vi "PNG Write.vi"(8 "error in (no error)":errorcluster, 10 "Chunks":T1[](array[typedef]) {"CRC" format="%08x"}, 11 "Image Path (*.png)":path) -> (0 "error out":errorcluster, 3 "dup Image Path":path)   [LabVIEW 2018, in "Export-Built-ins.lvlib"]
doc: "Writes the PNG image chunks to the <b>Image Path (*.png)</b>.\n\nCreated by: Ryan Pacini"
uses:
  Export-Built-ins.lvlib
  Controls/PNG Chunk.ctl
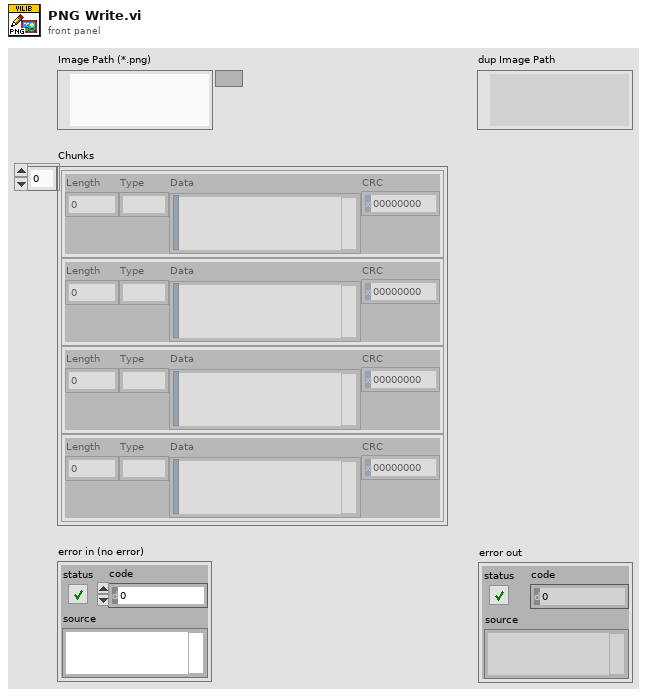
[diagram p1: front panel]
types:
  T1 = typedef "Export-Built-ins.lvlib/PNG Chunk.ctl" = cluster{"Length":i32, "Type":string, "Data":string, "CRC":u32}
  T2 = enum16{"open", "replace", "create", "open or create", "replace or create", "replace or create with confirmation"}
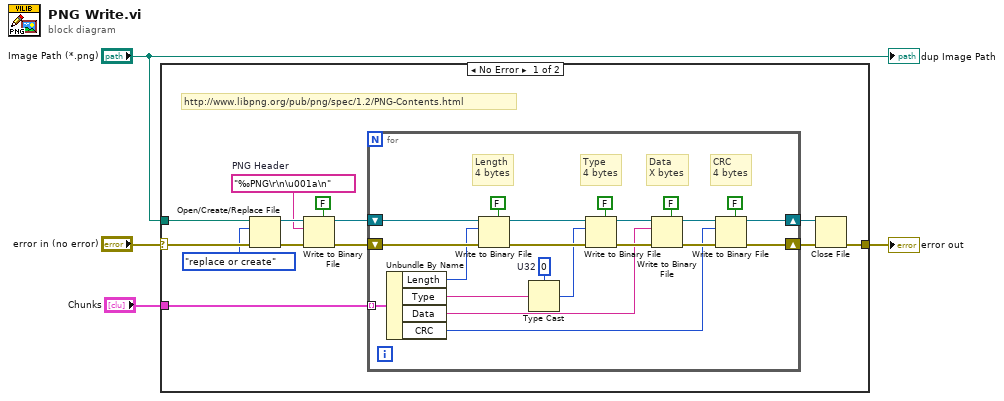
[diagram p0: block diagram]
diagram:
  n1 = case shown="No Error" "error in (no error)" {
    selector: "error in (no error)" -> [w17 w39]
    tunnel: "Image Path (*.png)" -> [w16 _]
    tunnel: [w13 w39] -> w3
    tunnel: "Chunks" -> [w5 _]
    frame No Error {
      w8 = "‰PNG\r\n\u001a\n"  # PNG Header
      # "http://www.libpng.org/pub/png/spec/1.2/PNG-Contents.html"
      n2 = Open/Create/Replace File(file path (use dialog)=w16, error in=w17, operation (0:open)=T2."replace or create") -> (refnum out=w15:refnum<file>, error out=w10:errorcluster)  [unwired: 3 in, 1 out]
      n3 = Write to Binary File(file (use dialog)=w15, data=w8, error in=w10, 5:FALSE ("prepend array or string size? (T)")) -> (refnum out=w7:refnum<file>, error out=w6:errorcluster)  [unwired: 2 in, 1 out]
      n4 = for {
        shift-right: [w19] -> w14
        shift-left: w6 -> [w35]
        tunnel: w5 -> [w38] mode=indexing
        shift-right: [w18] -> w12
        shift-left: w7 -> [w36]
        w29 = 0  # U32
        # "CRC\n4 bytes"
        # "Data\nX bytes"
        # "Type\n4 bytes"
        # "Length\n4 bytes"
        n5 = Unbundle By Name(w38) -> ("Length"=w34:i32, "Type"=w30:string, "Data"=w24:string, "CRC"=w20:u32)
        n6 = Write to Binary File(file (use dialog)=w36, data=w34, error in=w35, 5:FALSE ("prepend array or string size? (T)")) -> (refnum out=w31:refnum<file>, error out=w32:errorcluster)  [unwired: 2 in, 1 out]
        n7 = Type Cast(type=w29, x=w30) -> (*(type *) &x=w28:i32)
        n8 = Write to Binary File(file (use dialog)=w31, data=w28, error in=w32, 5:FALSE ("prepend array or string size? (T)")) -> (refnum out=w25:refnum<file>, error out=w26:errorcluster)  [unwired: 2 in, 1 out]
        n9 = Write to Binary File(file (use dialog)=w25, data=w24, error in=w26, 5:FALSE ("prepend array or string size? (T)")) -> (refnum out=w21:refnum<file>, error out=w22:errorcluster)  [unwired: 2 in, 1 out]
        n10 = Write to Binary File(file (use dialog)=w21, data=w20, error in=w22, 5:FALSE ("prepend array or string size? (T)")) -> (refnum out=w18:refnum<file>, error out=w19:errorcluster)  [unwired: 2 in, 1 out]
      }
      n11 = Close File(refnum=w12, error in=w14) -> (error out=w13:errorcluster)  [unwired: 1 out]
    }
    frame Error {
    }
  }
  "error out" <- w3
  "dup Image Path" <- "Image Path (*.png)"
